vi "CDL0100 Recipe Creator v1.0.vi"(0 "Previous Recipe Path":path=path "C:/ProgramData/TDK/CDL0100/Recipe.ini") -> (1 "New Recipe Path":path=path "C:/ProgramData/TDK/CDL0100/Recipe.ini", 2 "Rectifier Info Out":dbl[][](array[numeric]), 3 "canceled?":bool)   [LabVIEW 2019]
uses:
  <vilib>/Utility/config.llb/Write Key (Double).vi
  <vilib>/Utility/config.llb/Write Key (U32).vi
  <vilib>/Utility/config.llb/Read Key (Double).vi
  <vilib>/Utility/config.llb/Read Key (I32).vi
  <vilib>/Utility/config.llb/NI_LVConfig.lvlib
panel:
  out "Under100":string="! Sum < 100 !"
  out "Over100":string="! Sum > 100 !"
  in  "Constants":cluster{"F":dbl, "n":dbl, "r":dbl, "MW":dbl}={"F"=96485.0, "n"=2.0, "r"=8.95, "MW"=63.546}
  out "Total Amp Min":cluster{"Left (back)":dbl, "Right (front)":dbl}={"Left (back)"=1.15, "Right (front)"=1.15}
  in  "Frame Surface Area (dm^2)":cluster{"Left (back)":dbl, "Right (front)":dbl}={"Left (back)"=1.15, "Right (front)"=1.15}
  out "Plating Time":string
  out "Recipe Time\n(min)":dbl[][](array[numeric]) format="%#_4g"
  out "Rectifier Setpoints":dbl[][](array[numeric]) format="%.1f"
  in  "Plating Thickness (um)":cluster{"Left (back)":dbl, "Right (front)":dbl}
  in  "Surface Area (mm^2)":cluster{"Left (back)":dbl, "Right (front)":dbl}
  in  "Plating Steps":u32=1 min=1 max=5 step=1
  in  "New Version":i32
  in  "New Recipe Name":string
  in  "Recipe":dbl[][](array[numeric])
  in  "cancel":bool
  out "Previous Version":i32
  out "Previous Recipe Name":string
  in  "Save":bool
  # "LEFT (back)"
  # "RIGHT (front)"
  # "% of Plating"
  # "ASD"
  # "Amps"
  # "AmpMin"
  # "Amps"
  # "AmpMin"
  # "Left"
  # "Right"
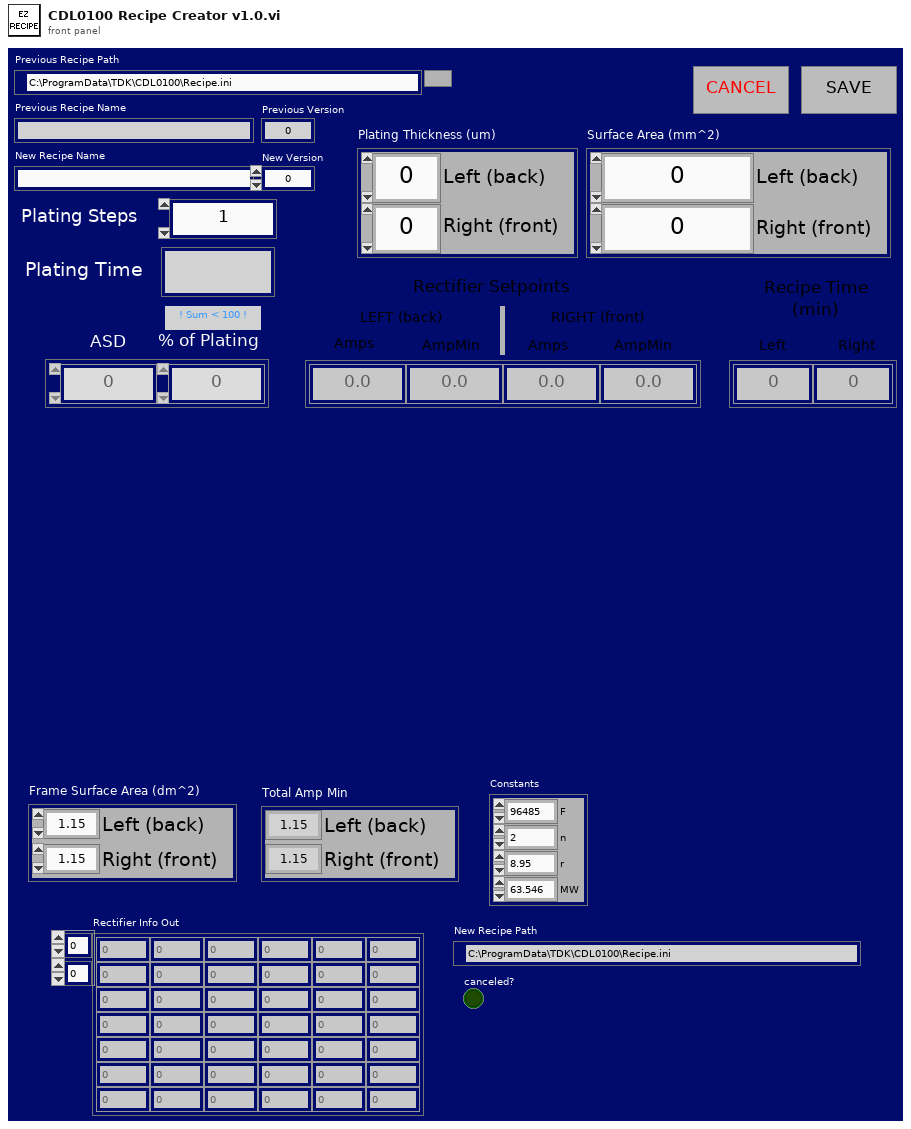
[diagram p1: front panel]
types:
  T1 = typedef "NI_LVConfig.lvlib/Config Data RefNum.ctl" = refnum<k1>
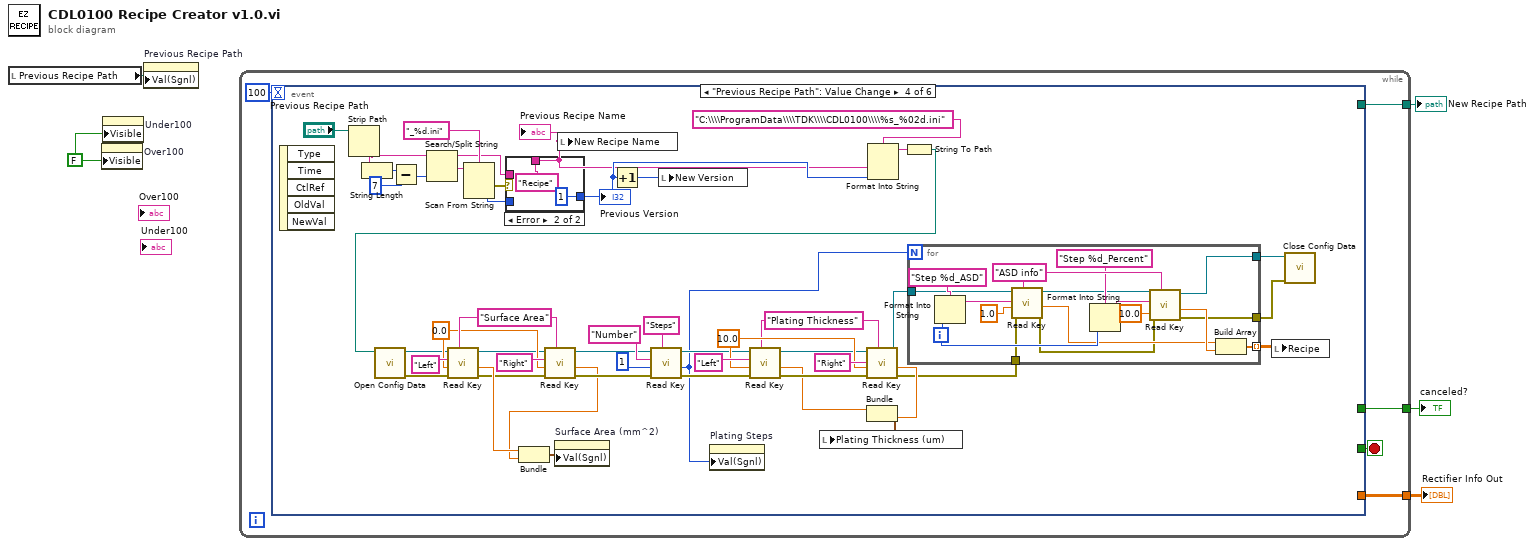
[diagram p0: block diagram]
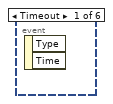
[diagram p2: hidden frame]
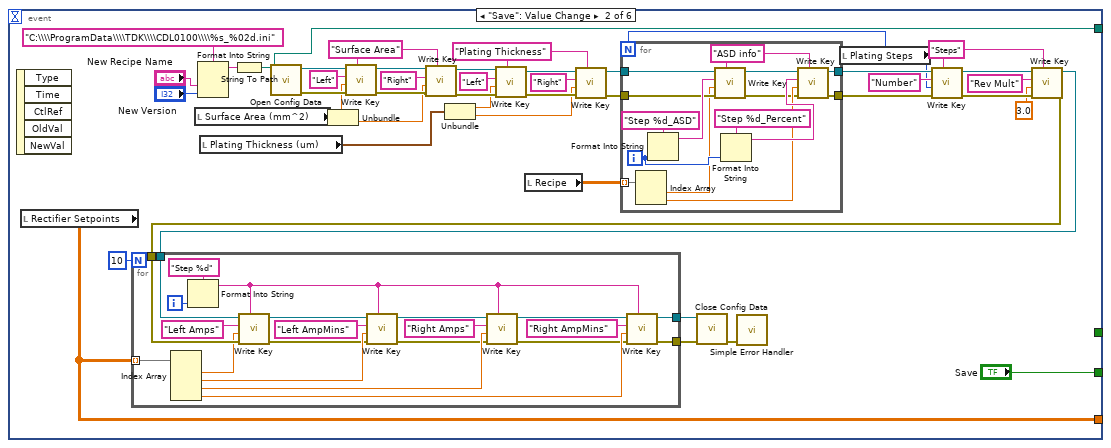
[diagram p3: hidden frame]
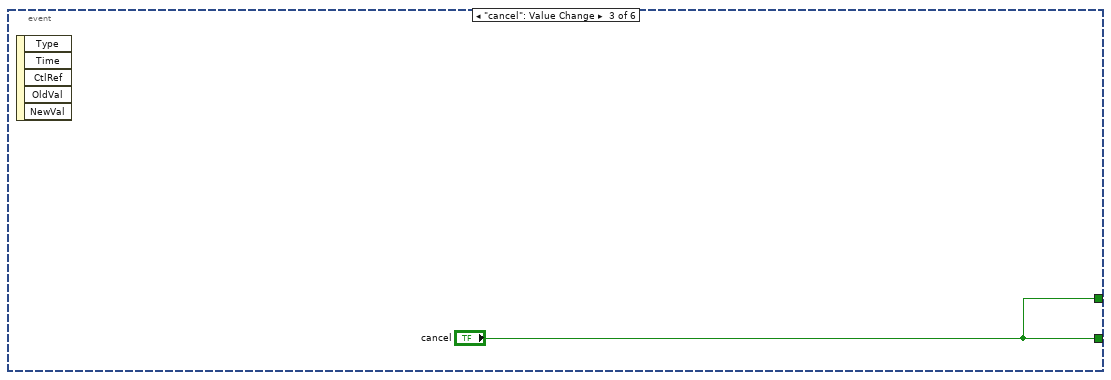
[diagram p4: hidden frame]
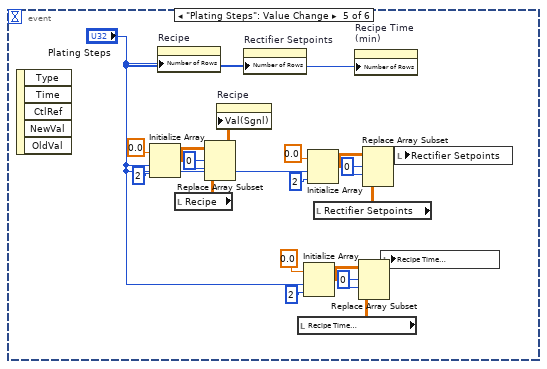
[diagram p6: hidden frame]
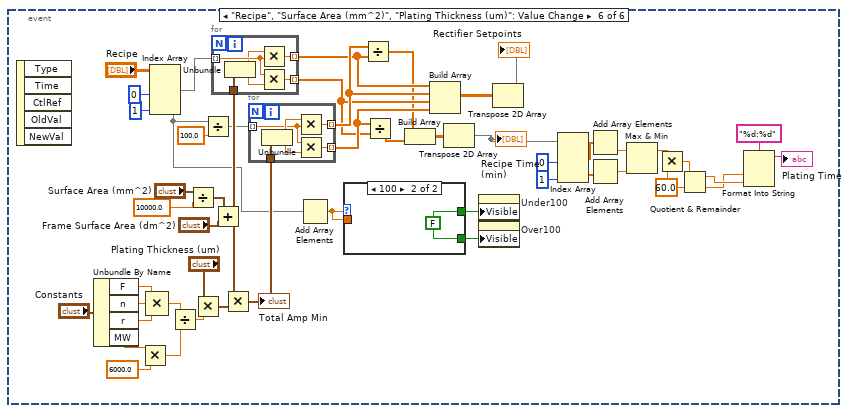
[diagram p7: hidden frame]
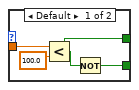
[diagram p8: hidden frame]
diagram:
  w1 = FALSE ("Visible")
  n1 = local read "Previous Recipe Path"() -> (w5:path)
  n2 = property on="Over100" class="Str"("Visible"=w1) -> ()  [unwired: 2 in, 2 out]
  n3 = property on="Under100" class="Str"("Visible"=w1) -> ()  [unwired: 2 in, 2 out]
  n4 = property on="Previous Recipe Path" class="Path"("Val(Sgnl)"=w5) -> ()  [unwired: 2 in, 2 out]
  n5 = while {
    tunnel: [w8] -> w4
    tunnel: [w7] -> w3
    tunnel: [w6] -> w2
    stop <- w10 stop-if-true
    n6 = event shown="[3] \"Previous Recipe Path\": Value Change" {
      selector: _ -> [_ _ _ _ _ _]
      dyn-events: _ -> [_ _ _ _ _ _]
      timeout: 100 -> [_ _ _ _ _ _]
      tunnel: [_ "Save" "cancel" _ _ _] -> w10
      tunnel: [_ w16 _ _ _ _] -> w8
      tunnel: [_ _ "cancel" _ _ _] -> w7
      tunnel: [_ w11 _ _ _ _] -> w6
      event Timeout {
        n7 = event-data() -> ()  [unwired: 1 in, 2 out]
      }
      event "Save": Value Change {
        w37 = "Plating Thickness" ("section")
        w17 = "Steps" ("section")
        w50 = "Surface Area" ("section")
        n8 = event-data() -> ()  [unwired: 1 in, 5 out]
        n9 = local read "Rectifier Setpoints"() -> (w16:dbl[][])
        n10 = local read "Surface Area (mm^2)"() -> (w46:cluster{"Left (back)":dbl, "Right (front)":dbl})
        n11 = Format Into String(format string="C:\\\\ProgramData\\\\TDK\\\\CDL0100\\\\%s_%02d.ini", "New Recipe Name", "New Version") -> (resulting string=w53:string)  [unwired: 2 in, 1 out]
        n12 = local read "Plating Thickness (um)"() -> (w30:cluster{"Left (back)":dbl, "Right (front)":dbl})
        n13 = String To Path(string=w53) -> (path=w11:path)
        n14 = call <vilib>:"Open Config Data.vi"("configuration file path"=w11) -> ("error out"=w51:errorcluster, "refnum"=w52:T1)  [unwired: 8 in, 1 out]
        n15 = Unbundle(w46) -> ("Left (back)"=w45:dbl, "Right (front)"=w44:dbl)
        n16 = call-poly <vilib>:"Write Key.vi"("section"=w50, "error in (no error)"=w51, "value"=w45, "key"="Left" ("section"), "refnum"=w52) -> ("error out"=w47:errorcluster, "refnum out"=w48:T1)  [unwired: 4 in, 1 out]
        n17 = call-poly <vilib>:"Write Key.vi"("section"=w50, "error in (no error)"=w47, "value"=w44, "key"="Right" ("section"), "refnum"=w48) -> ("error out"=w33:errorcluster, "refnum out"=w32:T1)  [unwired: 4 in, 1 out]
        n18 = Unbundle(w30) -> ("Left (back)"=w29:dbl, "Right (front)"=w28:dbl)
        n19 = call-poly <vilib>:"Write Key.vi"("section"=w37, "error in (no error)"=w33, "value"=w29, "key"="Left" ("section"), "refnum"=w32) -> ("error out"=w34:errorcluster, "refnum out"=w35:T1)  [unwired: 4 in, 1 out]
        n20 = local read "Recipe"() -> (w15:dbl[][])
        n21 = call-poly <vilib>:"Write Key.vi"("section"=w37, "error in (no error)"=w34, "value"=w28, "key"="Right" ("section"), "refnum"=w35) -> ("error out"=w26:errorcluster, "refnum out"=w27:T1)  [unwired: 4 in, 1 out]
        n22 = local read "Plating Steps"() -> (w23:u32)
        n23 = for {
          N: w23 -> [_]
          tunnel: w27 -> [w91]
          tunnel: w26 -> [w89]
          tunnel: w15 -> [w85] mode=indexing
          tunnel: [w79] -> w24
          tunnel: [w78] -> w25
          i -> [w88]
          w80 = "ASD info" ("format string")
          n24 = Index Array(array=w85) -> (element #1=w84:dbl, element #2=w83:dbl)  [unwired: 2 in]
          n25 = Format Into String(format string="Step %d_ASD", w88) -> (resulting string=w90:string)  [unwired: 2 in, 1 out]
          n26 = call-poly <vilib>:"Write Key.vi"("section"=w80, "error in (no error)"=w89, "value"=w84, "key"=w90, "refnum"=w91) -> ("error out"=w82:errorcluster, "refnum out"=w81:T1)  [unwired: 4 in, 1 out]
          n27 = Format Into String(format string="Step %d_Percent", w88) -> (resulting string=w86:string)  [unwired: 2 in, 1 out]
          n28 = call-poly <vilib>:"Write Key.vi"("section"=w80, "error in (no error)"=w82, "value"=w83, "key"=w86, "refnum"=w81) -> ("error out"=w79:errorcluster, "refnum out"=w78:T1)  [unwired: 4 in, 1 out]
        }
        n29 = call-poly <vilib>:"Write Key.vi"("section"=w17, "error in (no error)"=w24, "value"=w23, "key"="Number" ("section"), "refnum"=w25) -> ("error out"=w41:errorcluster, "refnum out"=w40:T1)  [unwired: 4 in, 1 out]
        n30 = call-poly <vilib>:"Write Key.vi"("section"=w17, "error in (no error)"=w41, "value"=3.0 ("Right (front)"), "key"="Rev Mult" ("section"), "refnum"=w40) -> ("error out"=w20:errorcluster, "refnum out"=w21:T1)  [unwired: 4 in, 1 out]
        n31 = for {
          N: 10 -> [_]
          tunnel: w16 -> [w77] mode=indexing
          tunnel: w21 -> [w76]
          tunnel: w20 -> [w75]
          tunnel: [w57] -> w19
          tunnel: [w56] -> w18
          i -> [w73]
          n32 = Index Array(array=w77) -> (element #1=w68:dbl, element #2=w63:dbl, element #3=w62:dbl, element #4=w61:dbl)  [unwired: 4 in]
          n33 = Format Into String(format string="Step %d", w73) -> (resulting string=w66:string)  [unwired: 2 in, 1 out]
          n34 = call-poly <vilib>:"Write Key.vi"("section"=w66, "error in (no error)"=w75, "value"=w68, "key"="Left Amps" ("format string"), "refnum"=w76) -> ("error out"=w58:errorcluster, "refnum out"=w71:T1)  [unwired: 4 in, 1 out]
          n35 = call-poly <vilib>:"Write Key.vi"("section"=w66, "error in (no error)"=w58, "value"=w63, "key"="Left AmpMins" ("format string"), "refnum"=w71) -> ("error out"=w59:errorcluster, "refnum out"=w70:T1)  [unwired: 4 in, 1 out]
          n36 = call-poly <vilib>:"Write Key.vi"("section"=w66, "error in (no error)"=w59, "value"=w62, "key"="Right Amps" ("format string"), "refnum"=w70) -> ("error out"=w60:errorcluster, "refnum out"=w69:T1)  [unwired: 4 in, 1 out]
          n37 = call-poly <vilib>:"Write Key.vi"("section"=w66, "error in (no error)"=w60, "value"=w61, "key"="Right AmpMins" ("format string"), "refnum"=w69) -> ("error out"=w57:errorcluster, "refnum out"=w56:T1)  [unwired: 4 in, 1 out]
        }
        n38 = call <vilib>:"Close Config Data.vi"("error in (no error)"=w19, "refnum"=w18) -> ("error out"=w14:errorcluster)  [unwired: 8 in, 1 out]
        n39 = call <vilib>:"Simple Error Handler.vi"("error in (no error)"=w14) -> ()  [unwired: 4 in, 5 out]
      }
      event "cancel": Value Change {
        n40 = event-data() -> ()  [unwired: 1 in, 5 out]
      }
      event "Previous Recipe Path": Value Change {
        w120 = 10.0 ("default value")
        w113 = 0.0 ("default value")
        w119 = "Plating Thickness" ("section")
        w114 = "Surface Area" ("section")
        n41 = event-data() -> ()  [unwired: 1 in, 5 out]
        n42 = Strip Path(path="Previous Recipe Path") -> (name=w142:string)  [unwired: 1 out]
        n43 = String Length(string=w142) -> (length=w141:i32)
        n44 = Subtract(x=w141, y=7) -> (x-y=w137:i32)
        n45 = Search/Split String(string=w142, offset (0)=w137) -> (substring before match=w135:string, match + rest of string=w139:string)  [unwired: 1 in, 1 out]
        n46 = Scan From String(format string="_%d.ini", input string=w139) -> (error out=w134:errorcluster, output 1=w136:i32)  [unwired: 3 in, 2 out]
        n47 = case shown="Error" w134 {
          tunnel: w136 -> [w160 _]
          tunnel: w135 -> [w161 _]
          tunnel: [w161 "Recipe" ("name")] -> w97
          tunnel: [w160 1] -> w98
          frame No Error {
          }
          frame Error {
          }
        }
        "Previous Recipe Name" <- w97
        "Previous Version" <- w98
        n48 = local write "New Recipe Name"(w97) -> ()
        n49 = Increment(x=w98) -> (x+1=w99:i32)
        n50 = local write "New Version"(w99) -> ()
        n51 = Format Into String(format string="C:\\\\ProgramData\\\\TDK\\\\CDL0100\\\\%s_%02d.ini", w97, w98) -> (resulting string=w100:string)  [unwired: 2 in, 1 out]
        n52 = String To Path(string=w100) -> (path=w94:path)
        n53 = call <vilib>:"Open Config Data.vi"("configuration file path"=w94) -> ("error out"=w102:errorcluster, "refnum"=w103:T1)  [unwired: 8 in, 1 out]
        n54 = call-poly <vilib>:"Read Key.vi"("section"=w114, "error in (no error)"=w102, "default value"=w113, "key"="Left", "refnum"=w103) -> ("error out"=w111:errorcluster, "value"=w131:dbl, "refnum out"=w112:T1)  [unwired: 3 in, 1 out]
        n55 = call-poly <vilib>:"Read Key.vi"("section"=w114, "error in (no error)"=w111, "default value"=w113, "key"="Right", "refnum"=w112) -> ("error out"=w110:errorcluster, "value"=w107:dbl, "refnum out"=w109:T1)  [unwired: 3 in, 1 out]
        n56 = Bundle("value"=w131, "value"=w107) -> (w130:cluster{"value":dbl, "value":dbl})  [unwired: 1 in]
        n57 = property on="Surface Area (mm^2)" class="Clust (strict)"("Val(Sgnl)"=w130) -> ()  [unwired: 2 in, 2 out]
        n58 = call-poly <vilib>:"Read Key.vi"("section"="Steps", "error in (no error)"=w110, "default value"=1 ("value"), "key"="Number", "refnum"=w109) -> ("error out"=w122:errorcluster, "value"=w106:i32, "refnum out"=w115:T1)  [unwired: 3 in, 1 out]
        n59 = property on="Plating Steps" class="DigNum (strict)"("Val(Sgnl)"=w106) -> ()  [unwired: 2 in, 2 out]
        n60 = call-poly <vilib>:"Read Key.vi"("section"=w119, "error in (no error)"=w122, "default value"=w120, "key"="Left", "refnum"=w115) -> ("error out"=w121:errorcluster, "value"=w117:dbl, "refnum out"=w118:T1)  [unwired: 3 in, 1 out]
        n61 = call-poly <vilib>:"Read Key.vi"("section"=w119, "error in (no error)"=w121, "default value"=w120, "key"="Right", "refnum"=w118) -> ("error out"=w104:errorcluster, "value"=w116:dbl, "refnum out"=w105:T1)  [unwired: 3 in, 1 out]
        n62 = Bundle("value"=w117, "value"=w116) -> (w124:cluster{"value":dbl, "value":dbl})  [unwired: 1 in]
        n63 = local write "Plating Thickness (um)"(w124) -> ()
        n64 = for {
          N: w106 -> [_]
          tunnel: [w149] -> w101 mode=indexing
          tunnel: [w147] -> w123
          tunnel: [w146] -> w108
          tunnel: w105 -> [w145]
          tunnel: w104 -> [w143]
          i -> [w155]
          w156 = "ASD info" ("section")
          n65 = Format Into String(format string="Step %d_ASD", w155) -> (resulting string=w158:string)  [unwired: 2 in, 1 out]
          n66 = call-poly <vilib>:"Read Key.vi"("section"=w156, "error in (no error)"=w143, "default value"=1.0, "key"=w158, "refnum"=w145) -> ("error out"=w148:errorcluster, "value"=w150:dbl, "refnum out"=w144:T1)  [unwired: 3 in, 1 out]
          n67 = Format Into String(format string="Step %d_Percent", w155) -> (resulting string=w153:string)  [unwired: 2 in, 1 out]
          n68 = call-poly <vilib>:"Read Key.vi"("section"=w156, "error in (no error)"=w148, "default value"=10.0, "key"=w153, "refnum"=w144) -> ("error out"=w147:errorcluster, "value"=w151:dbl, "refnum out"=w146:T1)  [unwired: 3 in, 1 out]
          n69 = Build Array(w150, w151) -> (w149:dbl[])
        }
        n70 = local write "Recipe"(w101) -> ()
        n71 = call <vilib>:"Close Config Data.vi"("error in (no error)"=w123, "refnum"=w108) -> ()  [unwired: 8 in, 2 out]
      }
      event "Plating Steps": Value Change {
        w170 = 0 ("index (row)")
        w177 = 0 ("index (row)")
        w179 = 0 ("index (row)")
        n72 = event-data() -> ()  [unwired: 1 in, 5 out]
        n73 = Initialize Array(0.0, "Plating Steps", 2 ("dimension size")) -> (w180:dbl[][])
        n74 = property on="Recipe" class="Arr (strict)"("Number of Rows"="Plating Steps") -> ()  [unwired: 2 in, 2 out]
        n75 = local read "Recipe"() -> (w178:dbl[][])
        n76 = Replace Array Subset(array=w180, new element=w178, index (row)=w179, index (col)=w179) -> (w164:dbl[][])
        n77 = property on="Recipe" class="Arr (strict)"("Val(Sgnl)"=w164) -> ()  [unwired: 2 in, 2 out]
        n78 = property on="Rectifier Setpoints" class="Arr (strict)"("Number of Rows"="Plating Steps") -> ()  [unwired: 2 in, 2 out]
        n79 = local read "Recipe Time\n(min)"() -> (w169:dbl[][])
        n80 = Initialize Array(0.0, "Plating Steps", 2 ("dimension size")) -> (w171:dbl[][])
        n81 = Initialize Array(0.0, "Plating Steps", 2 ("dimension size")) -> (w176:dbl[][])
        n82 = local read "Rectifier Setpoints"() -> (w166:dbl[][])
        n83 = property on="Recipe Time\n(min)" class="Arr (strict)"("Number of Rows"="Plating Steps") -> ()  [unwired: 2 in, 2 out]
        n84 = Replace Array Subset(array=w171, new element=w169, index (row)=w170, index (col)=w170) -> (w168:dbl[][])
        n85 = Replace Array Subset(array=w176, new element=w166, index (row)=w177, index (col)=w177) -> (w165:dbl[][])
        n86 = local write "Recipe Time\n(min)"(w168) -> ()
        n87 = local write "Rectifier Setpoints"(w165) -> ()
      }
      event "Recipe", "Surface Area (mm^2)", "Plating Thickness (um)": Value Change {
        w189 = 60.0 ("y")
        n88 = event-data() -> ()  [unwired: 1 in, 5 out]
        n89 = Unbundle By Name("Constants") -> ("F"=w227:dbl, "n"=w226:dbl, "r"=w225:dbl, "MW"=w224:dbl)
        n90 = Multiply(x=w224, y=6000.0) -> (x*y=w221:dbl)
        n91 = Compound Arithmetic op=MULTIPLY(w227, w226, w225) -> (w222:dbl)
        n92 = Index Array(array="Recipe", index (col) #1=0 ("disabled index (col)"), index (col) #2=1 ("index (col)")) -> (element #1=w216:dbl[], element #2=w184:dbl[])  [unwired: 2 in]
        n93 = Divide(x=w222, y=w221) -> (x/y=w219:dbl)
        n94 = Divide(x="Surface Area (mm^2)", y=10000.0) -> (x/y=w229:cluster{"Left (back)":dbl, "Right (front)":dbl})
        n95 = Multiply(x="Plating Thickness (um)", y=w219) -> (x*y=w218:cluster{"Left (back)":dbl, "Right (front)":dbl})
        n96 = Divide(x=w184, y=100.0) -> (x/y=w183:dbl[])
        n97 = Add(x=w229, y="Frame Surface Area (dm^2)") -> (x+y=w215:cluster{"Left (back)":dbl, "Right (front)":dbl})
        n98 = for {
          tunnel: w216 -> [w248] mode=indexing
          tunnel: w215 -> [w249]
          tunnel: [w245] -> w207 mode=indexing
          tunnel: [w244] -> w205 mode=indexing
          n99 = Unbundle(w249) -> ("Left (back)"=w246:dbl, "Right (front)"=w247:dbl)
          n100 = Multiply(x=w246, y=w248) -> (x*y=w245:dbl)
          n101 = Multiply(x=w248, y=w247) -> (x*y=w244:dbl)
        }
        n102 = Multiply(x=w215, y=w218) -> (x*y=w213:cluster{"Left (back)":dbl, "Right (front)":dbl})
        "Total Amp Min" <- w213
        n103 = for {
          tunnel: w183 -> [w238] mode=indexing
          tunnel: w213 -> [w243]
          tunnel: [w240] -> w208 mode=indexing
          tunnel: [w239] -> w206 mode=indexing
          n104 = Unbundle(w243) -> ("Left (back)"=w241:dbl, "Right (front)"=w242:dbl)
          n105 = Multiply(x=w241, y=w238) -> (x*y=w240:dbl)
          n106 = Multiply(x=w238, y=w242) -> (x*y=w239:dbl)
        }
        n107 = Add Array Elements(numeric array=w184) -> (sum=w187:dbl)
        n108 = case shown="100" w187 {
          tunnel: w187 -> [w236 _]
          tunnel: [w234 w237] -> w186
          tunnel: [w233 w237] -> w185
          frame Default {
            n109 = Less?(x=w236, y=100.0) -> (x < y?=w234:bool)
            n110 = Not(x=w234) -> (.not. x?=w233:bool)
          }
          frame 100 {
            w237 = FALSE ("Visible")
          }
        }
        n111 = Divide(x=w208, y=w207) -> (x/y=w204:dbl[])
        n112 = Divide(x=w206, y=w205) -> (x/y=w203:dbl[])
        n113 = Build Array(w204, w203) -> (w202:dbl[][])
        n114 = Build Array(w207, w208, w205, w206) -> (w210:dbl[][])
        n115 = Transpose 2D Array(2D array=w202) -> (transposed array=w201:dbl[][])
        "Recipe Time\n(min)" <- w201
        n116 = property on="Under100" class="Str"("Visible"=w186) -> ()  [unwired: 2 in, 2 out]
        n117 = property on="Over100" class="Str"("Visible"=w185) -> ()  [unwired: 2 in, 2 out]
        n118 = Transpose 2D Array(2D array=w210) -> (transposed array=→"Rectifier Setpoints":dbl[][])
        n119 = Index Array(array=w201, index (col) #1=0 ("disabled index (col)"), index (col) #2=1 ("index (col)")) -> (element #1=w197:dbl[], element #2=w198:dbl[])  [unwired: 2 in]
        n120 = Add Array Elements(numeric array=w197) -> (sum=w196:dbl)
        n121 = Add Array Elements(numeric array=w198) -> (sum=w195:dbl)
        n122 = Max & Min(x=w196, y=w195) -> (max(x,y)=w191:dbl)  [unwired: 1 out]
        n123 = Multiply(x=w191, y=w189) -> (x*y=w190:dbl)
        n124 = Quotient & Remainder(x=w190, y=w189) -> (x-y*floor(x/y)=w194:dbl, floor(x/y)=w188:dbl)
        n125 = Format Into String(format string="%d:%d" ("time format string (%c)"), w188, w194) -> (resulting string=→"Plating Time":string)  [unwired: 2 in, 1 out]
      }
    }
  }
  "Rectifier Info Out" <- w4
  "canceled?" <- w3
  "New Recipe Path" <- w2
